vi "11_21_Fxp_addation.vi"(1 "y":fxp<+/-,21,11>, 2 "x":fxp<+/-,21,11>) -> (0 "x+y":fxp<+/-,22,12> format="%.41g")   [LabVIEW 2020]
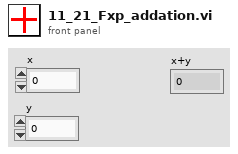
[diagram p1: front panel]
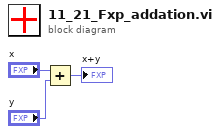
[diagram p0: block diagram]
diagram:
  n1 = Add(x="x", y="y") -> (x+y=→"x+y":fxp<+/-,22,12>)
